vi "draw_manual_overlay.vi"(8 "error in":errorcluster, 11 "Display State In":T1 {"array of overlays"."overlay size" min=1}) -> (0 "error out":errorcluster, 3 "Display State Out":T1 caption="State" {"array of overlays"."overlay size" min=1})   [LabVIEW 2010, in "XImage.xctl"]
uses:
  XImage.xctl
  state.ctl
  classes/SpaceVector/SpaceVector/SpaceVector.lvclass
  classes/PointCollection/PointCollection/PointCollection.lvclass
  ROI_frames_cluster.ctl
  control_refs_cluster.ctl
  calibration_cluster.ctl
  enumerations/unit.ctl
  xpath_cluster.ctl
  overlays_cluster.ctl
  ROI_mode_enum.ctl
  last_action_enum.ctl
  <vilib>/vision/Image Controls.llb/IMAQ Image.ctl
  classes/Image/Image/Image.lvclass
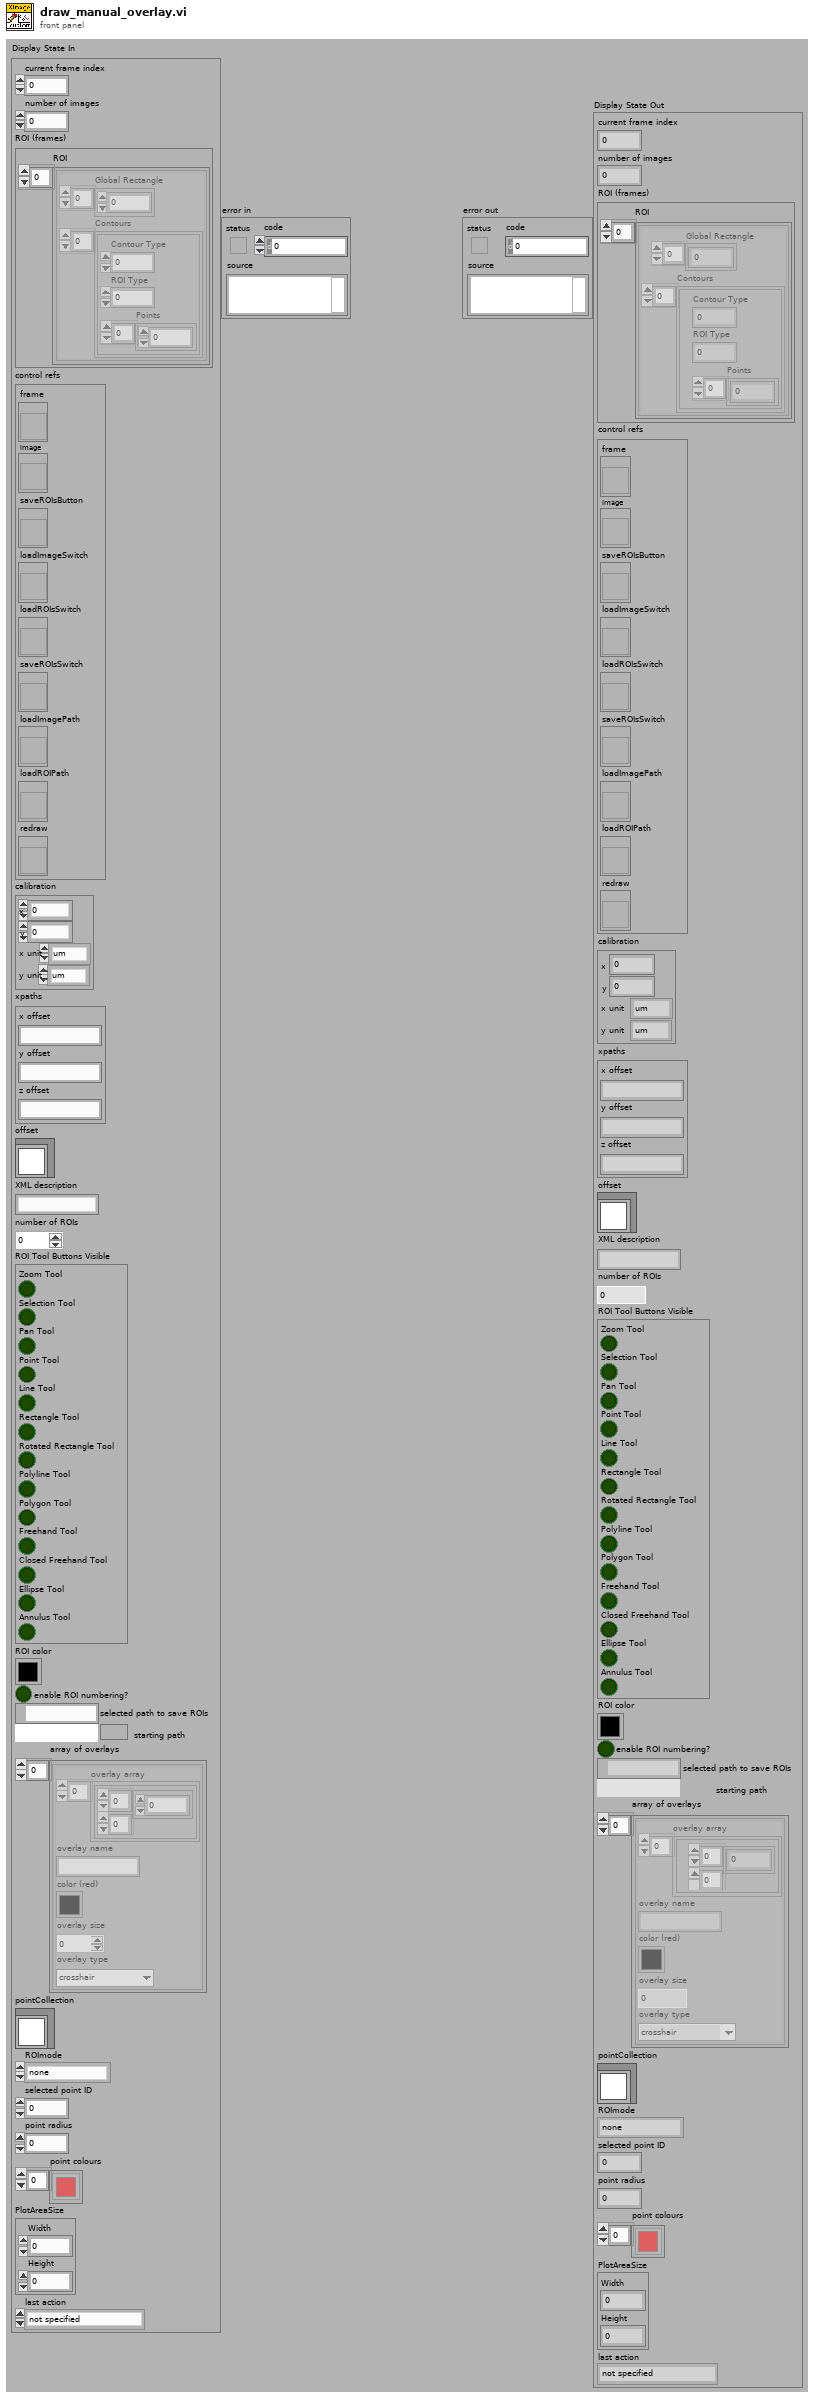
[diagram p1: front panel]
types:
  T1 = typedef "XImage.xctl/state.ctl" = cluster{"current frame index":i32, "number of images":i32, "ROI (frames)":T2, "control refs":T3, "calibration":T4, "xpaths":T6, "offset":refnum<class "SpaceVector.lvclass">, "XML description":string, "number of ROIs":dbl, "ROI Tool Buttons Visible":cluster{"Zoom Tool":bool, "Selection Tool":bool, "Pan Tool":bool, "Point Tool":bool, "Line Tool":bool, "Rectangle Tool":bool, "Rotated Rectangle Tool":bool, "Polyline Tool":bool, "Polygon Tool":bool, "Freehand Tool":bool, "Closed Freehand Tool":bool, "Ellipse Tool":bool, "Annulus Tool":bool}, "ROI color":u32, "enable ROI numbering?":bool, "selected path to save ROIs":path, "starting path":path, "array of overlays":T7[], "pointCollection":refnum<class "PointCollection.lvclass">, "ROImode":T8, "selected point ID":dbl, "point radius":i32, "point colours":u32[], "PlotAreaSize":cluster{"Width":u32, "Height":u32}, "last action":T9}
  T2 = typedef "XImage.xctl/ROI_frames_cluster.ctl" = cluster{"ROI":cluster{"Global Rectangle":i32[], "Contours":cluster{"Contour Type":u32, "ROI Type":u32, "Points":i32[]}[]}[]}
  T3 = typedef "XImage.xctl/control_refs_cluster.ctl" = cluster{"frame":refnum<vi>, "image":refnum<vi>, "saveROIsButton":refnum<vi>, "loadImageSwitch":refnum<vi>, "loadROIsSwitch":refnum<vi>, "saveROIsSwitch":refnum<vi>, "loadImagePath":refnum<vi>, "loadROIPath":refnum<vi>, "redraw":refnum<vi>}
  T4 = typedef "XImage.xctl/calibration_cluster.ctl" = cluster{"x":dbl, "y":dbl, "x unit":T5, "y unit":T5}
  T5 = typedef "Image.lvclass/unit.ctl" = enum16{"um", "s"}
  T6 = typedef "XImage.xctl/xpath_cluster.ctl" = cluster{"x offset":string, "y offset":string, "z offset":string}
  T7 = typedef "XImage.xctl/overlays_cluster.ctl" = cluster{"overlay array":cluster{i32[][]}[], "overlay name":string, "color (red)":u32, "overlay size":i32, "overlay type":enum16{"crosshair", "circle"}}
  T8 = typedef "XImage.xctl/ROI_mode_enum.ctl" = enum16{"none", "IMAQROIs", "PointCollection"}
  T9 = typedef "XImage.xctl/last_action_enum.ctl" = enum16{"not specified", "image loaded", "frame changed", "ROIs changed"}
  T10 = typedef "IMAQ Image.ctl" = refnum<image>
  T11 = cluster{"Left":i32, "Top":i32, "Right":i32, "Bottom":i32}
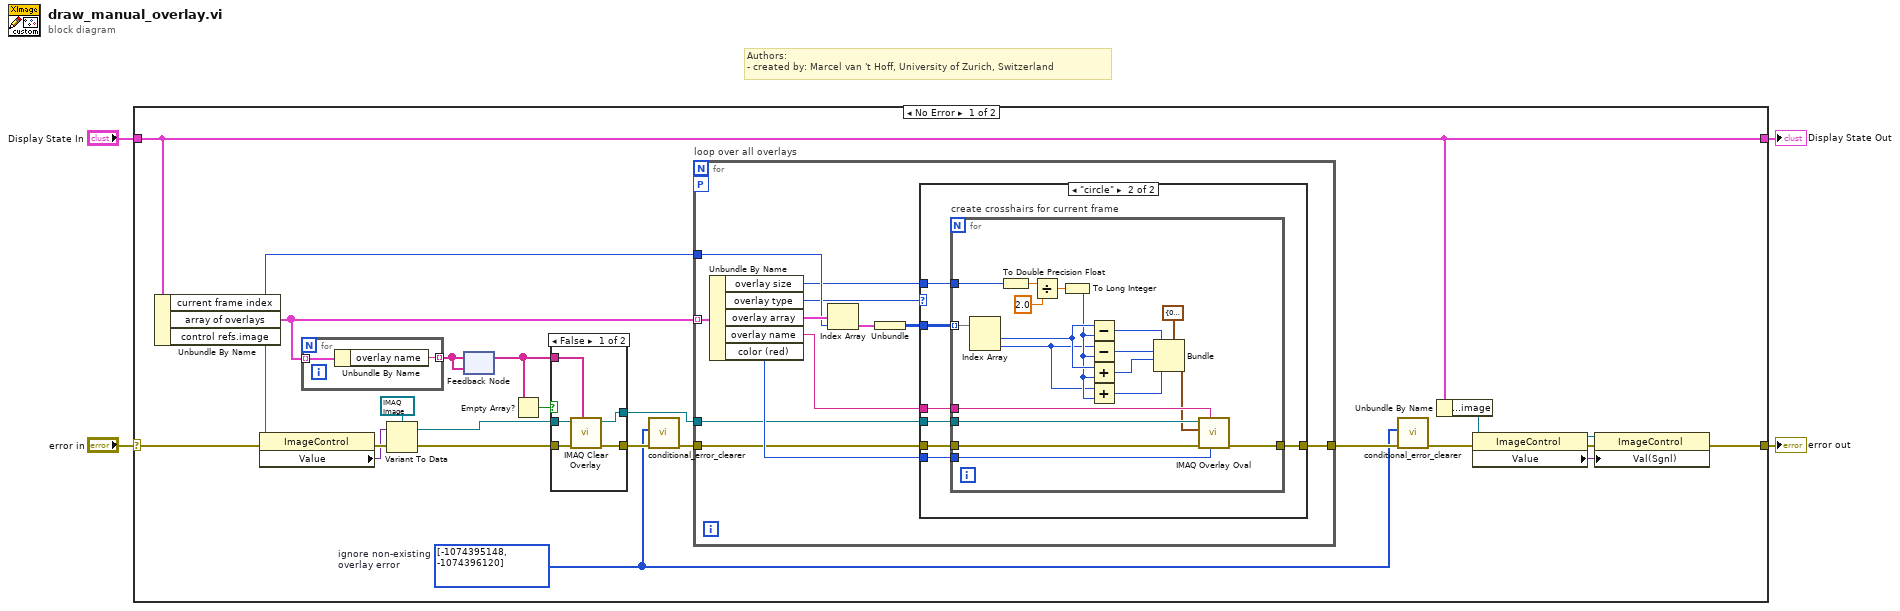
[diagram p0: block diagram]
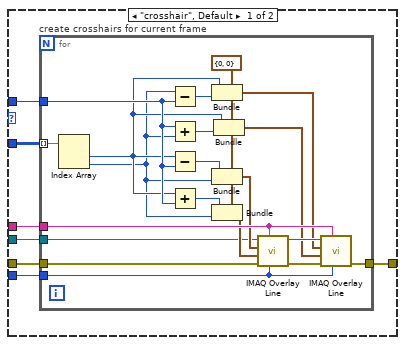
[diagram p3: hidden frame]
diagram:
  # "Authors: \n- created by: Marcel van 't Hoff, University of Zurich, Switzerland"
  n1 = case shown="No Error" "error in" {
    selector: "error in" -> [w28 w104]
    tunnel: "Display State In" -> [w18 w103]
    tunnel: [w19 w104] -> w2
    tunnel: [w18 w103] -> w1
    frame No Error {
      w13 = i32[] [-1074395148, -1074396120]  # ignore non-existing overlay error
      n2 = Unbundle By Name(w18) -> ("current frame index"=w24:i32, "array of overlays"=w20:T7[], "control refs.image"=w21:refnum<vi>)
      n3 = property class="ImageControl"(reference=w21, error in=w28) -> (error out=w27:errorcluster, "Value"=w26:variant)  [unwired: 1 out]
      n4 = for {
        tunnel: w20 -> [w102] mode=indexing
        tunnel: [w101] -> w7 mode=indexing
        n5 = Unbundle By Name(w102) -> ("overlay name"=w101:string)
      }
      n6 = Variant To Data(error in=w27, Variant=w26, type=T10 refnum ("New Image")) -> (error out=w23:errorcluster, data=w22:T10)
      n7 = feedback #1(w7) -> (w5:string[])
      n8 = feedback-in #1(w7) -> ()
      n9 = Empty Array?(array=w5) -> (empty?=w6:bool)
      n10 = case shown="False" w6 {
        tunnel: w23 -> [w33 w35]
        tunnel: w22 -> [w32 w34]
        tunnel: [w31 w34] -> w16
        tunnel: [w30 w35] -> w15
        tunnel: w5 -> [w29 _]
        frame False {
          n11 = call "IMAQ Clear Overlay"("Groups"=w29, "error in (no error)"=w33, "Image"=w32) -> ("error out"=w30:errorcluster, "Image Out"=w31:T10)  [unwired: 7 in]
        }
        frame True {
        }
      }
      n12 = call "conditional_error_clearer.vi"("error in (no error)"=w15, "array of clearable error codes"=w13) -> ("error out"=w14:errorcluster)  [unwired: 9 in]
      n13 = for "loop over all overlays" {
        tunnel: w20 -> [w43] mode=indexing
        tunnel: w24 -> [w42]
        tunnel: w14 -> [w39]
        tunnel: [w41] -> w17
        tunnel: w16 -> [w40]
        workers-P: _ -> [_]
        n14 = Unbundle By Name(w43) -> ("overlay size"=w37:i32, "overlay type"=w36:enum16{"crosshair", "circle"}, "overlay array"=w47:cluster{i32[][]}[], "overlay name"=w38:string, "color (red)"=w44:u32)
        n15 = Index Array(array=w47, index=w42) -> (element=w46:cluster{i32[][]})
        n16 = Unbundle(w46) -> (w45:i32[][])
        n17 = case shown="\"circle\"" w36 {
          tunnel: w45 -> [w54 w81]
          tunnel: w44 -> [w53 w80]
          tunnel: [w52 w79] -> w41
          tunnel: w40 -> [w51 w78]
          tunnel: w39 -> [w50 w77]
          tunnel: w38 -> [w49 w76]
          tunnel: w37 -> [w48 w75]
          frame "crosshair", Default {
            n18 = for "create crosshairs for current frame" {
              tunnel: w54 -> [w67] mode=indexing
              tunnel: w53 -> [w70]
              tunnel: w49 -> [w71]
              tunnel: w48 -> [w61]
              tunnel: w50 -> [w59]
              tunnel: [w72] -> w52
              tunnel: w51 -> [w58]
              w57 = cluster{"X":i32, "Y":i32} {"X"=0, "Y"=0} ("Origin")
              n19 = Index Array(array=w67) -> (element #1=w56:i32, element #2=w55:i32)  [unwired: 2 in]
              n20 = Subtract(x=w55, y=w61) -> (x-y=w62:i32)
              n21 = Add(x=w61, y=w55) -> (x+y=w60:i32)
              n22 = Subtract(x=w56, y=w61) -> (x-y=w63:i32)
              n23 = Add(x=w56, y=w61) -> (x+y=w64:i32)
              n24 = Bundle(cluster=w57, "X"=w56, "Y"=w62) -> (w66:cluster{"X":i32, "Y":i32})
              n25 = Bundle(cluster=w57, "X"=w63, "Y"=w55) -> (w69:cluster{"X":i32, "Y":i32})
              n26 = Bundle(cluster=w57, "X"=w64, "Y"=w55) -> (w68:cluster{"X":i32, "Y":i32})
              n27 = Bundle(cluster=w57, "X"=w56, "Y"=w60) -> (w65:cluster{"X":i32, "Y":i32})
              n28 = call "IMAQ Overlay Line"("Color"=w70, "Group"=w71, "error in (no error)"=w59, "End Point"=w68, "Start Point"=w69, "Image"=w58) -> ("error out"=w73:errorcluster, "Image Out"=w74:T10)  [unwired: 4 in]
              n29 = call "IMAQ Overlay Line"("Color"=w70, "Group"=w71, "error in (no error)"=w73, "End Point"=w65, "Start Point"=w66, "Image"=w74) -> ("error out"=w72:errorcluster)  [unwired: 4 in, 1 out]
            }
          }
          frame "circle" {
            n30 = for "create crosshairs for current frame" {
              tunnel: w81 -> [w100] mode=indexing
              tunnel: w80 -> [w97]
              tunnel: w76 -> [w98]
              tunnel: w75 -> [w92]
              tunnel: w77 -> [w95]
              tunnel: [w99] -> w79
              tunnel: w78 -> [w96]
              n31 = Index Array(array=w100) -> (element #1=w87:i32, element #2=w84:i32)  [unwired: 2 in]
              n32 = To Double Precision Float(number=w92) -> (double precision float=w90:dbl)
              n33 = Divide(x=w90, y=2.0) -> (x/y=w89:dbl)
              n34 = To Long Integer(number=w89) -> (32bit integer=w85:i32)
              n35 = Subtract(x=w87, y=w85) -> (x-y=w88:i32)
              n36 = Subtract(x=w84, y=w85) -> (x-y=w82:i32)
              n37 = Add(x=w87, y=w85) -> (x+y=w86:i32)
              n38 = Add(x=w84, y=w85) -> (x+y=w83:i32)
              n39 = Bundle(cluster=T11 {"Left"=0, "Top"=0, "Right"=0, "Bottom"=0} ("Bounding Rectangle"), "Left"=w88, "Top"=w82, "Right"=w86, "Bottom"=w83) -> (w94:T11)
              n40 = call "IMAQ Overlay Oval"("Color"=w97, "Group"=w98, "error in (no error)"=w95, "Bounding Rectangle"=w94, "Image"=w96) -> ("error out"=w99:errorcluster)  [unwired: 5 in, 1 out]
            }
          }
        }
      }
      n41 = call "conditional_error_clearer.vi"("error in (no error)"=w17, "array of clearable error codes"=w13) -> ("error out"=w8:errorcluster)  [unwired: 9 in]
      n42 = Unbundle By Name(w18) -> ("control refs.image"=w12:refnum<vi>)
      n43 = property class="ImageControl"(reference=w12, error in=w8) -> (reference out=w11:refnum<vi>, error out=w10:errorcluster, "Value"=w9:variant)
      n44 = property class="ImageControl"(reference=w11, error in=w10, "Val(Sgnl)"=w9) -> (error out=w19:errorcluster)  [unwired: 1 out]
    }
    frame Error {
    }
  }
  "error out" <- w2
  "Display State Out" <- w1
